vi "subStage_CalcGridPos.vi"(7 "Grid step size (mm)":dbl[](array[numeric])=[0.22186666666666666, 0.22186666666666666], 8 "error in (no error)":errorcluster, 9 "Yj":i32, 10 "Xi":i32, 11 "XY scan":T2={"XY scan?"=FALSE, "YY/XX"=[1, 1], "X0Y0"=[65.7434, 45.179, 0.0]}) -> (0 "error out":errorcluster, 3 "Stage-Ctrl":T1={"Console"={"L"=FALSE, "R"=FALSE, "FWD"=FALSE, "BACK"=FALSE}, "Step Width [mm]"=1.0, "Destination [mm]"=[6.0, 7.0], "Move "=FALSE} {"Destination [mm]" format="%_6g"; "Step Width [mm]" min=0.0 format="%_6f"})   [LabVIEW 2015]
panel:
  # "X"
  # "Y"
  # "Lengthwise"
  # "Crosswise"
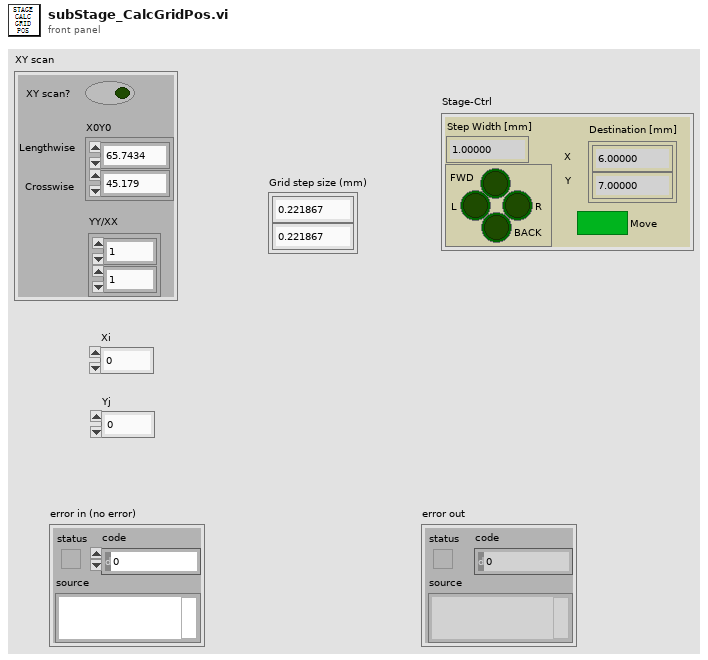
[diagram p1: front panel]
types:
  T1 = cluster{"Console":cluster{"L":bool, "R":bool, "FWD":bool, "BACK":bool}, "Step Width [mm]":dbl, "Destination [mm]":dbl[], "Move ":bool}
  T2 = cluster{"XY scan?":bool, "YY/XX":i32[], "X0Y0":dbl[]}
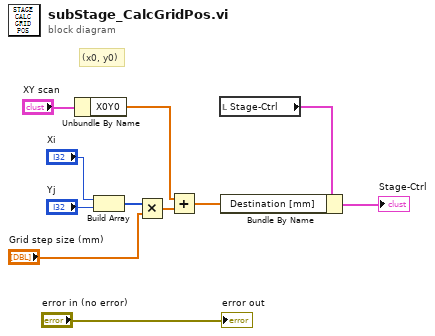
[diagram p0: block diagram]
diagram:
  # "(x0, y0)"
  n1 = Unbundle By Name("XY scan") -> ("X0Y0"=w4:dbl[])
  n2 = Build Array("Xi", "Yj") -> (w9:i32[])
  n3 = Multiply(x=w9, y="Grid step size (mm)") -> (x*y=w7:dbl[])
  n4 = Add(x=w4, y=w7) -> (x+y=w2:dbl[])
  n5 = local read "Stage-Ctrl"() -> (w3:T1)
  n6 = Bundle By Name(cluster=w3, "Destination [mm]"=w2) -> (→"Stage-Ctrl":T1)
  "error out" <- "error in (no error)"
